vi "LadrcProjMain.vi"() -> ()   [LabVIEW 2018]
panel:
  out "y/dt":dbl
  out "y":dbl
  out "波形图表":cluster{"排水速度":dbl, "控制量 u":dbl}(graph)
  out "z1":dbl
  out "z2":dbl
  out "z3":dbl
  out "u 2":dbl
  out "out":dbl
  out "y+z1":cluster{"y(k+1)":dbl, "z1(k+1)":dbl}(graph)
  out "dy/dt+z2":cluster{dbl, dbl}(graph)
  out "u":dbl(graph)
  out "水池水位":dbl(slide) scale=0.0..1.2
  in  "排水速度":dbl(slide)=0.3 scale=0.0..1.0
  out "进水速度-自动":dbl(slide) scale=-2.0..2.0
  in  "控制量 u":dbl format="%.3f"
  # "+"
  # "R"
  # "kp"
  # "OUT1"
  # "+"
  # "对象"
  # "u"
  # "+"
  # "1/b0"
  # "-"
  # "-"
  # "白线：实际y\n红线：ESO"
  # "y"
  # "kd"
  # "z3"
  # "z2"
  # "线性扩张\n状态观测器"
  # "z1"
  # "LESO"
  # "白色实际\n红色z"
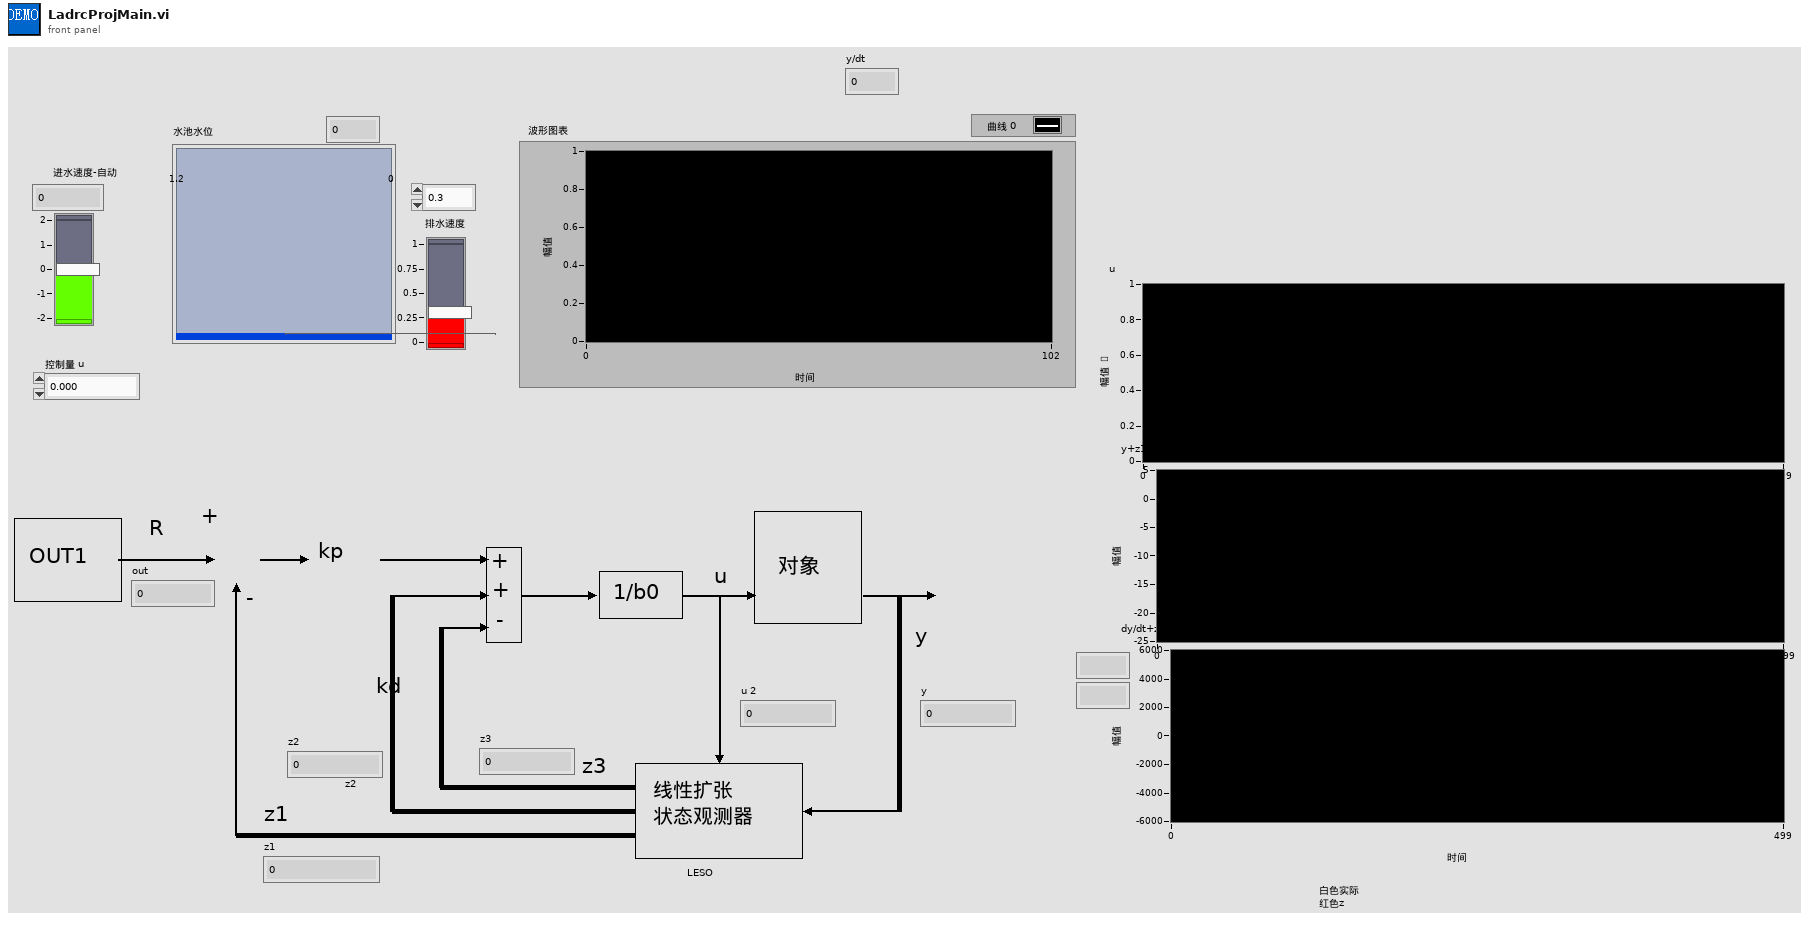
[diagram p1: front panel]
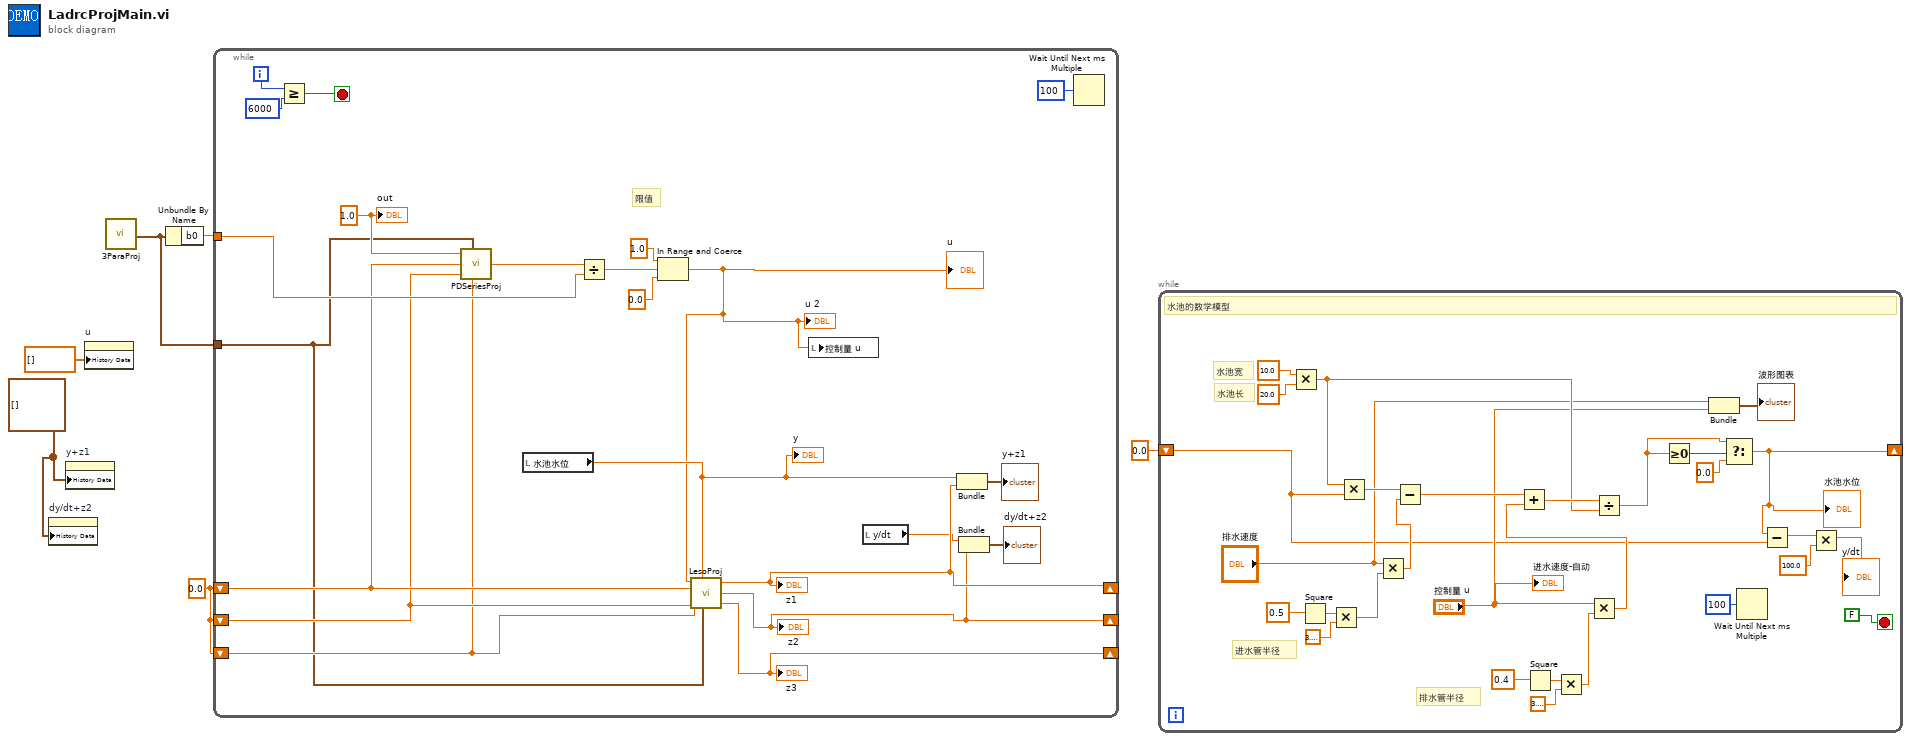
[diagram p0: block diagram]
diagram:
  w4 = cluster{dbl, dbl}[] [] ("历史数据")
  w5 = 0.0 ("z1(k+1)")
  n1 = property on="dy/dt+z2" class="WFChart (严格)"("History Data"=w4) -> ()  [unwired: 2 in, 2 out]
  n2 = property on="y+z1" class="WFChart (严格)"("History Data"=w4) -> ()  [unwired: 2 in, 2 out]
  n3 = property on="u" class="WFChart (严格)"("History Data"=dbl[] [] ("历史数据")) -> ()  [unwired: 2 in, 2 out]
  n4 = call "3ParaProj.vi"() -> ("3Parameter"=w1:cluster{"b0":dbl, "w0":dbl, "wc":dbl})
  n5 = Unbundle By Name(w1) -> ("b0"=w2:dbl)
  n6 = while {
    tunnel: w2 -> [w27]
    shift-right: [w24] -> _
    shift-left: w5 -> [w11]
    shift-right: [w23] -> _
    shift-left: w5 -> [w10]
    shift-right: [w22] -> _
    shift-left: w5 -> [w9]
    tunnel: w1 -> [w7]
    i -> [w18]
    stop <- w25 stop-if-true
    w12 = 1.0 ("x")
    # "限值"
    n7 = Greater Or Equal?(x=w18, y=6000) -> (x >= y?=w25:bool)
    n8 = call "PDSeriesProj.vi"("Input"=w12, "3Parameter"=w7, "Z1"=w11, "Z2"=w10, "Z3"=w9) -> ("U0-Z3"=w8:dbl)
    n9 = local read "水池水位"() -> (w19:dbl)
    "y" <- w19
    n10 = Divide(x=w8, y=w27) -> (x/y=w16:dbl)
    n11 = In Range and Coerce(upper limit=1.0 ("上限"), x=w16, lower limit=0.0 ("下限")) -> (coerced(x)=w15:dbl)  [unwired: 1 out]
    "u 2" <- w15
    "u" <- w15
    n12 = call "LesoProj.vi"("u"=w15, "y"=w19, "z1(k)"=w11, "z3(k)"=w9, "3Parameter"=w7, "z2(k)"=w10) -> ("z1(k+1)"=w24:dbl, "z2(k+1)"=w23:dbl, "z3(k+1)"=w22:dbl)
    "z1" <- w24
    "z2" <- w23
    "z3" <- w22
    n13 = local write "控制量 u"(w15) -> ()
    n14 = local read "y/dt"() -> (w17:dbl)
    n15 = Bundle("水池水位"=w19, "z1(k+1)"=w24) -> (→"y+z1":cluster{"水池水位":dbl, "z1(k+1)":dbl})  [unwired: 1 in]
    n16 = Bundle("y/dt"=w17, "z2(k+1)"=w23) -> (→"dy/dt+z2":cluster{"y/dt":dbl, "z2(k+1)":dbl})  [unwired: 1 in]
    n17 = Wait Until Next ms Multiple(millisecond multiple=u32 100 ("毫秒倍数")) -> ()  [unwired: 1 out]
    "out" <- w12
  }
  n18 = while {
    shift-right: [w33] -> _
    shift-left: 0.0 -> [w32]
    stop <- FALSE stop-if-true
    # "排水管半径"
    # "进水管半径"
    # "水池宽"
    # "水池长"
    # "水池的数学模型"
    n19 = Multiply(x=10.0 ("y"), y=20.0) -> (x*y=w40:dbl)
    n20 = Square(x=0.5) -> (x^2=w52:dbl)
    n21 = Multiply(x=w52, y=3.141592653589793) -> (x*y=w51:dbl)
    n22 = Multiply(x=w40, y=w32) -> (x*y=w54:dbl)
    n23 = Multiply(x="排水速度", y=w51) -> (x*y=w53:dbl)
    n24 = Subtract(x=w54, y=w53) -> (x-y=w48:dbl)
    n25 = Square(x=0.4) -> (x^2=w44:dbl)
    n26 = Multiply(x=w44, y=3.141592653589793) -> (x*y=w45:dbl)
    n27 = Multiply(x="控制量 u", y=w45) -> (x*y=w43:dbl)
    n28 = Add(x=w48, y=w43) -> (x+y=w41:dbl)
    n29 = Divide(x=w41, y=w40) -> (x/y=w36:dbl)
    n30 = Greater Or Equal To 0?(x=w36) -> (x >= 0?=w37:bool)
    n31 = Bundle("排水速度"="排水速度", "控制量 u"="控制量 u") -> (→"波形图表":cluster{"排水速度":dbl, "控制量 u":dbl})  [unwired: 1 out]
    n32 = Select(t=w36, s=w37, f=0.0) -> (s? t:f=w33:dbl)
    "水池水位" <- w33
    n33 = Wait Until Next ms Multiple(millisecond multiple=u32 100) -> ()  [unwired: 1 out]
    n34 = Subtract(x=w33, y=w32) -> (x-y=w30:dbl)
    n35 = Multiply(x=w30, y=100.0) -> (x*y=→"y/dt":dbl)
    "进水速度-自动" <- "控制量 u"
  }
